vi "#242.vi"   [LabVIEW 2017]
uses:
  user.lib/_NEVSTOP/Communicable State Machine(CSM)/_Support/Priority Queue/Priority Queue.lvclass/Priority Queue.ctl
  user.lib/_NEVSTOP/Communicable State Machine(CSM)/Utility/Build Error Cluster.vi
  user.lib/_NEVSTOP/Communicable State Machine(CSM)/_Support/Process/CSMP-Sync Call.vi
  user.lib/_NEVSTOP/Communicable State Machine(CSM)/Utility/uuid.vi
  user.lib/_NEVSTOP/Communicable State Machine(CSM)/Utility/Trim Both Whitespace.vi
  user.lib/_NEVSTOP/Communicable State Machine(CSM)/_Support/CSMQ/_CSMObj-Message Check.vi
  user.lib/_NEVSTOP/Communicable State Machine(CSM)/_Support/CSMQ/_CSMObj-Enqueue Cross-Module Message.vi
  user.lib/_NEVSTOP/Communicable State Machine(CSM)/_Support/CSMQ/_CSMOFGV Get.vi
  user.lib/_NEVSTOP/Communicable State Machine(CSM)/_Support/Priority Queue/Enqueue Element.vi
  user.lib/_NEVSTOP/Communicable State Machine(CSM)/_Support/CSMQ/_CSMOFGV.vi
  user.lib/_NEVSTOP/Communicable State Machine(CSM)/Communicable State Machine.lvlib
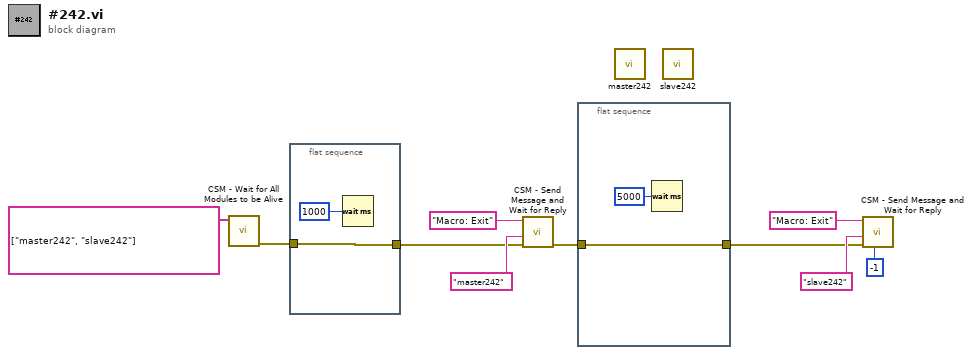
[diagram p0: block diagram]
diagram:
  n1 = call "CSM - Wait for All Modules to be Alive.vi"("Module Names (in)"=string[] ["master242", "slave242"]) -> ("Error out"=w1:errorcluster)  [unwired: 8 in, 2 out]
  n2 = flat-sequence {
    tunnel: [w11] -> w2
    tunnel: w1 -> [w11]
    frame #0 {
      n3 = Wait (ms)(milliseconds to wait=u32 1000) -> ()  [unwired: 1 out]
    }
  }
  n4 = call "CSM - Send Message and Wait for Reply.vi"("Error In (no error)"=w2, "Target Module"="master242", "State"="Macro: Exit") -> ("error out"=w4:errorcluster)  [unwired: 6 in, 2 out]
  n5 = flat-sequence {
    tunnel: [w13] -> w5
    tunnel: w4 -> [w13]
    frame #0 {
      n6 = Wait (ms)(milliseconds to wait=u32 5000) -> ()  [unwired: 1 out]
    }
  }
  n7 = call "master242.vi"() -> ()  [unwired: 12 in]
  n8 = call "slave242.vi"() -> ()  [unwired: 12 in]
  n9 = call "CSM - Send Message and Wait for Reply.vi"("Response Timeout(5000ms)"=-1, "Error In (no error)"=w5, "Target Module"="slave242", "State"="Macro: Exit") -> ()  [unwired: 5 in, 3 out]
